vi "Auto Warmup Shooter.vi"(11 "Shot Type":i32) -> ()   [LabVIEW 2015]
uses:
  Common Code/Shooter Commands.ctl
  Common Code/Shoot Modes Enum.ctl
  Common Code/Shot Type.ctl
  Common Code/Drivetrain Modes.ctl
  Robot Global Data.vi
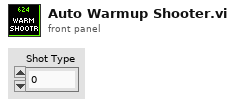
[diagram p1: front panel]
types:
  T1 = typedef "Shoot Modes Enum.ctl" = enum16{"Manual", "Safe", "Auto"}
  T2 = typedef "Shooter Commands.ctl" = enum16{"Idle", "Prime Shooter", "Shoot"}
  T3 = typedef "Drivetrain Commands.ctl" = cluster{"Y Power":dbl, "Turn Power":dbl, "1st Gear?":bool, "Modes":T4, "Heading Target":dbl, "X Max Speed":dbl, "Y Max Speed":dbl, "X Min Speed":dbl, "Y Min Speed":dbl, "Y Target":dbl, "Max Accel":dbl, "Max Velocity":dbl, "Y Power 2":dbl, "Pivot Speed":dbl}
  T4 = typedef "Drivetrain Modes.ctl" = enum16{"Tank", "Climb", "Manual", "Goal Vision Targeting", "PID Distance Drive", "Hybrid", "Gyro Steer"}
  T5 = typedef "Shooter Command Cluster.ctl" = cluster{"Command":T2, "Mode":T1, "Shot Type":T6, "Override Trigger Sensor":bool, "Override Angle?":bool, "Hide From Death":bool}
  T6 = typedef "Shot Type.ctl" = enum16{"Batter Shot", "Corner Shot", "Curve Shot", "Vision Shot", "Deep Middle Shot"}
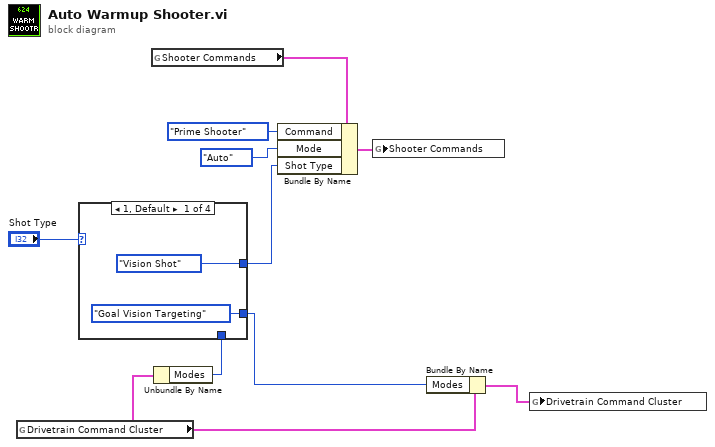
[diagram p0: block diagram]
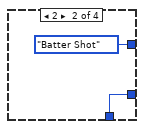
[diagram p2: hidden frame]
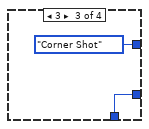
[diagram p3: hidden frame]
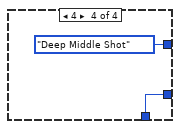
[diagram p4: hidden frame]
diagram:
  n1 = global read "Robot Global Data.vi" "Drivetrain Command Cluster"() -> (w3:T3)
  n2 = global read "Robot Global Data.vi" "Shooter Commands"() -> (w8:T5)
  n3 = Unbundle By Name(w3) -> ("Modes"=w2:T4)
  n4 = case shown="1, Default" "Shot Type" {
    tunnel: [Shot_Type."Vision Shot" ("Shot Type") Shot_Type."Batter Shot" ("Shot Type") Shot_Type."Corner Shot" ("Shot Type") Shot_Type."Deep Middle Shot" ("Shot Type")] -> w7
    tunnel: w2 -> [_ w13 w15 w17]
    tunnel: [Drivetrain_Modes."Goal Vision Targeting" ("Modes") w13 w15 w17] -> w1
    frame 1, Default {
    }
    frame 2 {
    }
    frame 3 {
    }
    frame 4 {
    }
  }
  n5 = Bundle By Name(cluster=w8, "Command"=Shooter_Commands."Prime Shooter", "Mode"=Shoot_Modes_Enum."Auto", "Shot Type"=w7) -> (w9:T5)
  n6 = global write "Robot Global Data.vi" "Shooter Commands"(w9) -> ()
  n7 = Bundle By Name(cluster=w3, "Modes"=w1) -> (w4:T3)
  n8 = global write "Robot Global Data.vi" "Drivetrain Command Cluster"(w4) -> ()
